vi "move_without_loop.vi"(0 "X":dbl, 1 "i":i32, 2 "run":bool, 5 "Y":dbl, 7 "deg":dbl, 9 "speed":dbl, 11 "offset":dbl format="%#_13g", 12 "dt":dbl) -> (4 "speed out":dbl[](array[numeric]), 10 "t2?":bool, 13 "speed out single":dbl, 14 "rotate speed":dbl, 15 "complet":bool)   [LabVIEW 2019]
panel:
  out "t3":dbl
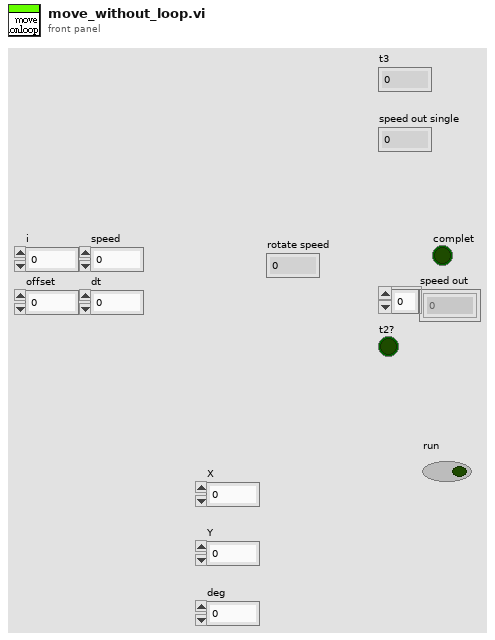
[diagram p1: front panel]
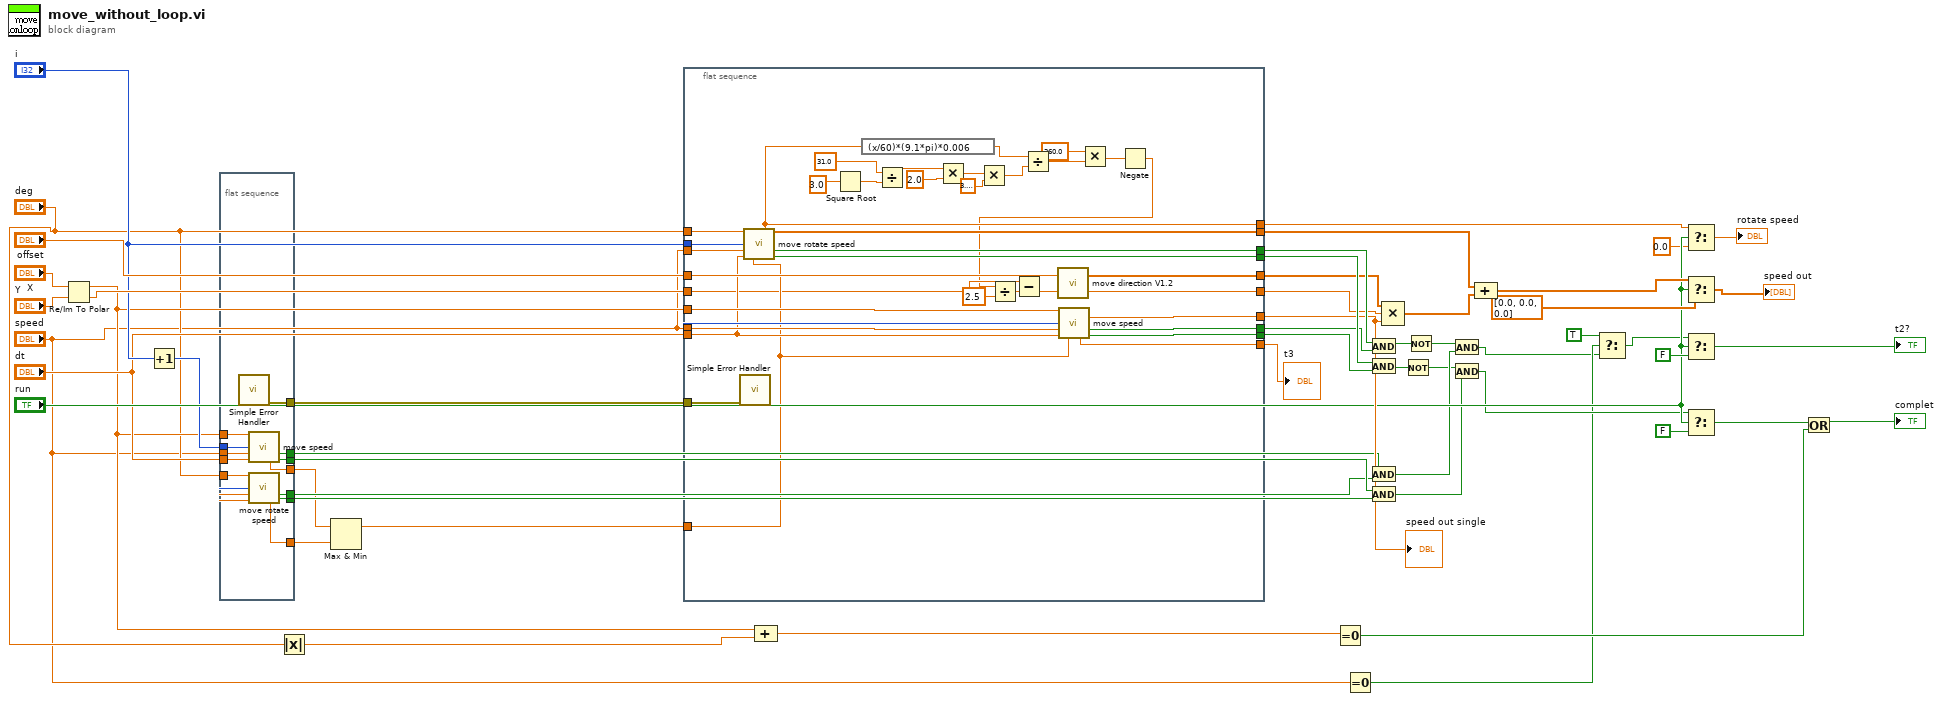
[diagram p0: block diagram]
diagram:
  n1 = Re/Im To Polar(2:"Y", 3:"X") -> (0:w42:dbl, 1:w14:dbl)
  n2 = Increment(x="i") -> (x+1=w30:i32)
  n3 = flat-sequence {
    tunnel: w30 -> [w66]
    tunnel: "speed" -> [w65]
    tunnel: "deg" -> [w64]
    tunnel: w14 -> [w63]
    tunnel: "dt" -> [w62]
    tunnel: [w61] -> w28
    tunnel: [w60] -> w27
    tunnel: [w59] -> w26
    tunnel: [w58] -> w25
    tunnel: [w57] -> w17
    tunnel: [w56] -> w4
    tunnel: [w55] -> w5
    frame #0 {
      n4 = call <vilib>:"Simple Error Handler.vi"() -> ("error out"=w57:errorcluster)  [unwired: 5 in, 4 out]
      n5 = call "move speed.vi"("X"=w63, "i"=w66, "speed"=w65, "dt(s)"=w62) -> ("t2?"=w58:bool, "t3"=w56:dbl, "complet?"=w60:bool)  [unwired: 7 in, 2 out]
      n6 = call "move rotate speed.vi"("rotate degree"=w64, "i"=w66, "speed"=w65, "dt(s)"=w62) -> ("t2?"=w59:bool, "t3"=w55:dbl, "complet?"=w61:bool)  [unwired: 5 in, 4 out]
    }
  }
  n7 = Absolute Value(x="deg") -> (abs(x)=w15:dbl)
  n8 = Max & Min(x=w4, y=w5) -> (max(x,y)=w2:dbl)  [unwired: 1 out]
  n9 = flat-sequence {
    tunnel: [w102] -> w54
    tunnel: [w101] -> w53
    tunnel: [w100] -> w52
    tunnel: [w99] -> w51
    tunnel: [w98] -> w50
    tunnel: [w97] -> w49
    tunnel: [w96] -> w48
    tunnel: [w95] -> w46
    tunnel: "offset" -> [w94]
    tunnel: w42 -> [w70]
    tunnel: [w72] -> w33
    tunnel: "i" -> [w93]
    tunnel: "speed" -> [w92]
    tunnel: "deg" -> [w91]
    tunnel: w14 -> [w90]
    tunnel: "dt" -> [w88]
    tunnel: w17 -> [w89]
    tunnel: "speed" -> [w87]
    tunnel: w2 -> [w86]
    tunnel: [w85] -> w1
    frame #0 {
      n10 = call <vilib>:"Simple Error Handler.vi"("error in (no error)"=w89) -> ()  [unwired: 4 in, 5 out]
      n11 = call "move rotate speed.vi"("rotate degree"=w91, "i"=w93, "speed"=w87, "dt(s)"=w88, "t3 in"=w86) -> ("speed"=w72:dbl, "speed out"=w95:dbl[], "t2?"=w100:bool, "complet?"=w102:bool)  [unwired: 4 in, 3 out]
      n12 = Square Root(x=3.0) -> (sqrt(x)=w83:dbl)
      n13 = expression code="(x/60)*(9.1*pi)*0.006"(w72) -> (w75:dbl)
      n14 = Divide(x=31.0, y=w83) -> (x/y=w81:dbl)
      n15 = Multiply(x=w81, y=2.0) -> (x*y=w78:dbl)
      n16 = Multiply(x=w78, y=3.141592653589793) -> (x*y=w76:dbl)
      n17 = Divide(x=w75, y=w76) -> (x/y=w77:dbl)
      n18 = call "move speed.vi"("X"=w90, "i"=w93, "speed"=w92, "dt(s)"=w88, "t3 in"=w86) -> ("speed out"=w97:dbl, "t2?"=w99:bool, "t3"=w85:dbl, "complet?"=w101:bool)  [unwired: 6 in, 1 out]
      n19 = Multiply(x=360.0, y=w77) -> (x*y=w74:dbl)
      n20 = Negate(x=w74) -> (-x=w68:dbl)
      n21 = Divide(x=w68, y=2.5) -> (x/y=w69:dbl)
      n22 = Subtract(x=w70, y=w69) -> (x-y=w71:dbl)
      n23 = call "move direction V1.2.vi"("theta"=w71, "offset"=w94) -> ("max value"=w96:dbl, "out array"=w98:dbl[])
    }
  }
  n24 = Compound Arithmetic op=ADD(w14, w15) -> (w12:dbl)
  n25 = Equal To 0?(x=w12) -> (x = 0?=w11:bool)
  n26 = Equal To 0?(x="speed") -> (x = 0?=w10:bool)
  n27 = And(x=w52, y=w51) -> (x .and. y?=w24:bool)
  n28 = And(x=w54, y=w53) -> (x .and. y?=w22:bool)
  n29 = And(x=w25, y=w26) -> (x .and. y?=w23:bool)
  n30 = And(x=w27, y=w28) -> (x .and. y?=w21:bool)
  n31 = Compound Arithmetic op=MULTIPLY(w50, w48, w49) -> (w47:dbl[])
  n32 = Not(x=w22) -> (.not. x?=w18:bool)
  n33 = Not(x=w24) -> (.not. x?=w19:bool)
  n34 = And(x=w19, y=w23) -> (x .and. y?=w6:bool)
  n35 = And(x=w18, y=w21) -> (x .and. y?=w20:bool)
  n36 = Compound Arithmetic op=ADD(w46, w47) -> (w38:dbl[])
  n37 = Select(t=TRUE, s=w10, f=w6) -> (s? t:f=w8:bool)
  n38 = Select(t=w33, s="run", f=0.0) -> (s? t:f=→"rotate speed":dbl)
  n39 = Select(t=w38, s="run", f=dbl[] [0.0, 0.0, 0.0]) -> (s? t:f=→"speed out":dbl[])
  n40 = Select(t=w8, s="run", f=FALSE) -> (s? t:f=→"t2?":bool)
  n41 = Select(t=w20, s="run", f=FALSE) -> (s? t:f=w41:bool)
  n42 = Or(x=w41, y=w11) -> (x .or. y?=→"complet":bool)
  "speed out single" <- w49
  "t3" <- w1
